vi "FGV - KH Gain.vi"(4 "error in":errorcluster, 6 "Function":enum16{"write", "read"}(ring), 7 "Gains":dbl[](array[numeric])) -> (0 "error out":errorcluster, 3 "Gains":dbl[](array[numeric]))   [LabVIEW 2016, in "KH7008.lvclass"]
uses:
  KH7008.lvclass
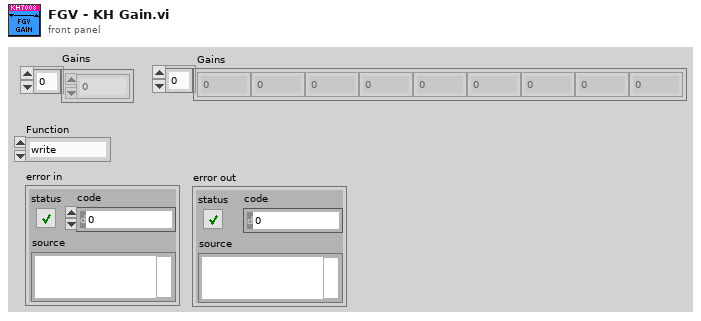
[diagram p1: front panel]
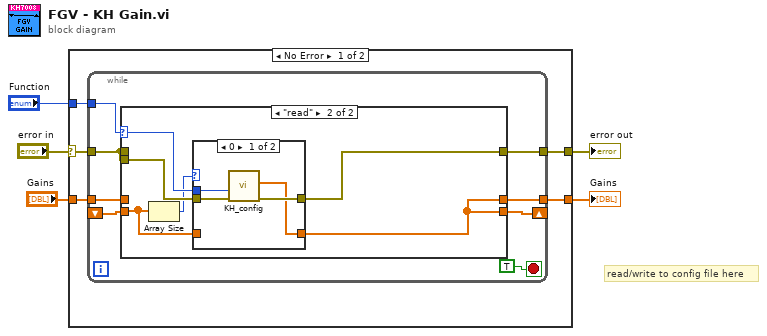
[diagram p0: block diagram]
diagram:
  # "read/write to config file here"
  n1 = case shown="No Error" "error in" {
    selector: "error in" -> [w10 w34]
    tunnel: [w9 w34] -> w4
    tunnel: "Gains" -> [w8 w33]
    tunnel: [w7 w33] -> w2
    tunnel: "Function" -> [w6 _]
    frame No Error {
      n2 = while {
        shift-right: [w13] -> _
        shift-left: _ -> [w12]
        tunnel: w10 -> [w11]
        tunnel: [w17] -> w9
        tunnel: w8 -> [w16]
        tunnel: [w15] -> w7
        tunnel: w6 -> [w14]
        stop <- TRUE stop-if-true
        n3 = case shown="\"read\"" w14 {
          selector: w14 -> [_ w26]
          tunnel: w11 -> [w19 _]
          tunnel: [w19 w24] -> w17
          tunnel: w16 -> [w20 _]
          tunnel: [w20 w22] -> w15
          tunnel: [w20 w22] -> w13
          tunnel: w12 -> [_ w21]
          tunnel: w11 -> [_ w25]
          frame "write", Default {
          }
          frame "read" {
            n4 = Array Size(array=w21) -> (size(s)=w23:i32)
            n5 = case shown="0" w23 {
              tunnel: w26 -> [w30 _]
              tunnel: w25 -> [w29 w32]
              tunnel: [w28 w32] -> w24
              tunnel: [w27 w31] -> w22
              tunnel: w21 -> [_ w31]
              frame 0 {
                n6 = call "KH_config.vi"("Error In"=w29, "Function"=w30) -> ("Error Out"=w28:errorcluster, "Gains out"=w27:dbl[])  [unwired: 7 in, 1 out]
              }
              frame 1, Default {
              }
            }
          }
        }
      }
    }
    frame Error {
    }
  }
  "error out" <- w4
  "Gains" <- w2
